vi "Measure Output Values.vi"(8 "error in (no error)":errorcluster, 10 "Wait Before Query (1550 ms)":u32=1550, 11 "VISA resource name":refnum<visa-resource-name>) -> (0 "error out":errorcluster, 1 "Current Output":dbl, 2 "Voltage Output":dbl, 3 "VISA resource name out":refnum<visa-resource-name>)   [LabVIEW 2023]
doc: "Measures the output voltage and current."
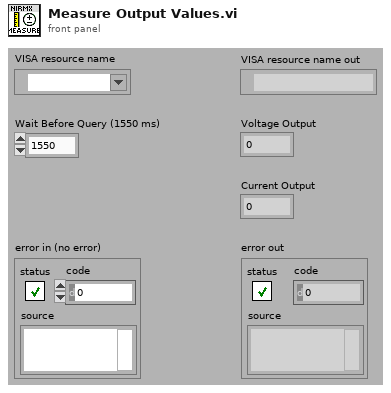
[diagram p1: front panel]
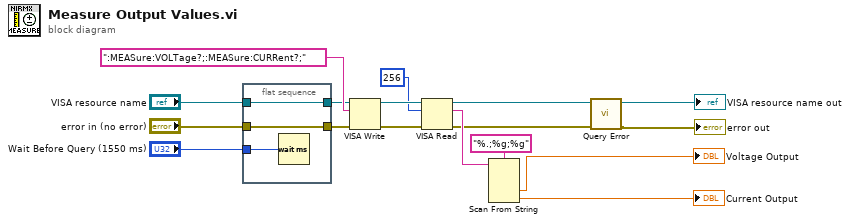
[diagram p0: block diagram]
diagram:
  n1 = flat-sequence {
    tunnel: "Wait Before Query (1550 ms)" -> [w20]
    tunnel: "VISA resource name" -> [w19]
    tunnel: [w19] -> w8
    tunnel: "error in (no error)" -> [w18]
    tunnel: [w18] -> w6
    frame #0 {
      n2 = Wait (ms)(milliseconds to wait=w20) -> ()  [unwired: 1 out]
    }
  }
  n3 = VISA Write(VISA resource name=w8, write buffer=":MEASure:VOLTage?;:MEASure:CURRent?;", error in (no error)=w6) -> (VISA resource name out=w15:refnum<visa-resource-name>, error out=w16:errorcluster)  [unwired: 1 out]
  n4 = VISA Read(VISA resource name=w15, byte count=u32 256, error in (no error)=w16) -> (VISA resource name out=w1:refnum<visa-resource-name>, read buffer=w14:string, error out=w2:errorcluster)  [unwired: 1 out]
  n5 = Scan From String(format string="%.;%g;%g", input string=w14) -> (output 1=→"Voltage Output":dbl, output 2=→"Current Output":dbl)  [unwired: 4 in, 3 out]
  n6 = call "Query Error.vi"("error in (no error)"=w2, "VISA resource name"=w1) -> ("error out"=→"error out":errorcluster, "VISA resource name out"=→"VISA resource name out":refnum<visa-resource-name>)  [unwired: 6 in, 2 out]
